vi "Write Attributes Metadata.vi"(7 "Actor in":refnum<class "Actor.lvclass">, 10 "Attributes Metadata":refnum<class "Attributes Metadata.lvclass">) -> (5 "Actor out":refnum<class "Actor.lvclass">)   [LabVIEW 2020, in "jettl.lvlib"]
uses:
  jettl.lvlib
  Actor/Actor.lvclass
  Attributes Metadata/Attributes Metadata.lvclass
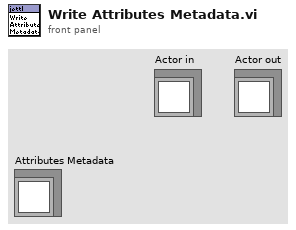
[diagram p1: front panel]
types:
  T1 = typedef "jettl.lvlib/Attributes.ctl" = cluster{"Unified Msgs":T2, "Unified Leaf":bool, "Edge Actors":refnum<class "Actor.lvclass">[], "Core Actors":refnum<class "Actor.lvclass">[], "Root":bool, "Alias":string, "UID":i32, "Transport":refnum<class "Transport.lvclass">, "This VI":refnum<vi>, "Attributes Metadata":refnum<class "Attributes Metadata.lvclass">, "Post-Setup Actors":refnum<class "Actor.lvclass">[]}
  T2 = typedef "jettl.lvlib/Msgs.ctl" = set{refnum<class "Msg.lvclass">}
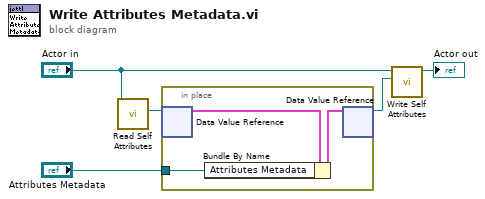
[diagram p0: block diagram]
diagram:
  n1 = call-dynamic "Read Self Attributes.vi"("Actor in"="Actor in") -> ("Self Attributes"=w3:refnum<data-value>)  [unwired: 10 in]
  n2 = in-place {
    in-place-border: "Attributes Metadata" -> [w6]
    n3 = in-place-dvr #1(w3) -> (w8:T1)  [unwired: 1 out]
    n4 = Bundle By Name(cluster=w8, "Attributes Metadata"=w6) -> (w7:T1)
    n5 = in-place-dvr #1(w7) -> (w2:refnum<data-value>)  [unwired: 1 out]
  }
  n6 = call-dynamic "Write Self Attributes.vi"("Self Attributes"=w2, "Actor in"="Actor in") -> ("Actor out"=→"Actor out":refnum<class "Actor.lvclass">)  [unwired: 9 in]
